vi "Basic_pn_SH.vi"(7 "BitFile Path":string="C:\\Users\\kalyan\\Desktop\\5775_digitizer\\Host\\PXIe_5775_KU035.lvbitx", 9 "AI num samples":u64=320 step=16, 10 "AI channels":string="AI0,AI1", 11 "Device Id":string="PXI1Slot5") -> (0 "error out":errorcluster, 1 "dt":dbl, 2 "SecondChannel":dbl[](array[numeric]), 3 "FirstChannel":dbl[](array[numeric]))   [LabVIEW 2019, in "GettingStarted_5775_Host.lvlib"]
uses:
  GettingStarted_5775_Host.lvlib
  <instrlib>/FlexRIO/API/Host/v1/NI FlexRIO/API/Reference Clock Source.ctl
  <instrlib>/FlexRIO/API/Host/v1/NI FlexRIO/API/Configure Reference Clock.vi
  <instrlib>/FlexRIO/API/Host/v1/NI FlexRIO/API/Get Property Reference - Fpga Small.vi
  <instrlib>/FlexRIO/API/Host/v1/NI FlexRIO/API/Configure Analog Start Trigger.vi
  <instrlib>/FlexRIO/API/Host/v1/NI FlexRIO/API/Configure Digital Edge Start Trigger.vi
  <instrlib>/FlexRIO/API/Host/v1/NI FlexRIO/API/Configure Immediate Start Trigger.vi
  <instrlib>/FlexRIO/API/Host/v1/NI FlexRIO/API/Read Stream 2D F64.vi
  <vilib>/FPGAPlugInAG/Dynamic/niLvFpga_Close_Dynamic.vi
  <vilib>/rvi/interface/nirviCloseFPGA/nirviCloseFPGA.xnode
  <instrlib>/FlexRIO/API/Host/v1/NI FlexRIO API v1.lvlib
  <resource>/objmgr/niflexrioapiStream.rc
panel:
  out "numSamples":i32
  in  "reference clock source":T1 items=["Default", "Onboard", "PXI_Clk10", "External", "None", "Baseboard Reference"]
  out "Acquisition time":dbl=3200000000.0 format="%#_6p"
  in  "ADC Interleaving Factor":i32=1 min=0 max=2 step=1
  out "Device Power":dbl(slide) scale=-1.0..38.0 scale format="%#_3p"
  out "FPGA Temperature":dbl(slide) scale=0.0..100.0 scale format="%#_3p"
  in  "Trigger Type":enum32{"Immediate", "Analog", "Digital"}(tab)
  in  "trigger channel":string="AI0"
  in  "rising edge?":bool=TRUE
  in  "level (V)":dbl format="%#_3p"
  in  "hysteresis (V)":dbl format="%#_3p"
  in  "digital trigger source":string(combo)
  in  "Waveform Tab Control":enum32{"AI Time Domain", "AI Frequency Domain"}(tab)
  out "Waveform Graph":dbl[][](graph)
  out "Limit (W)":dbl
  out "Power (W)":dbl
  out "Limit (C)":dbl
  out "Temp (C)":dbl format="%#_4p"
  # "Overview: Configure an acquisition for a FlexRIO target and transfer the data to the host using the FlexRIO Host API.  Loop an output waveform\nRequirements: FlexRIO\nInstructions: \n 1. Select the RIO Device that corresponds to the FlexRIO target. \n 2. Select the bitfile path that corresponds to your device\n 3. Optionally configure the clocking, stream, and trigger. \n 4. Run the VI"
  # "Resource Configuration"
  # "Clocking configuration"
  # "Input Waveform Configuration"
  # "Device Monitoring"
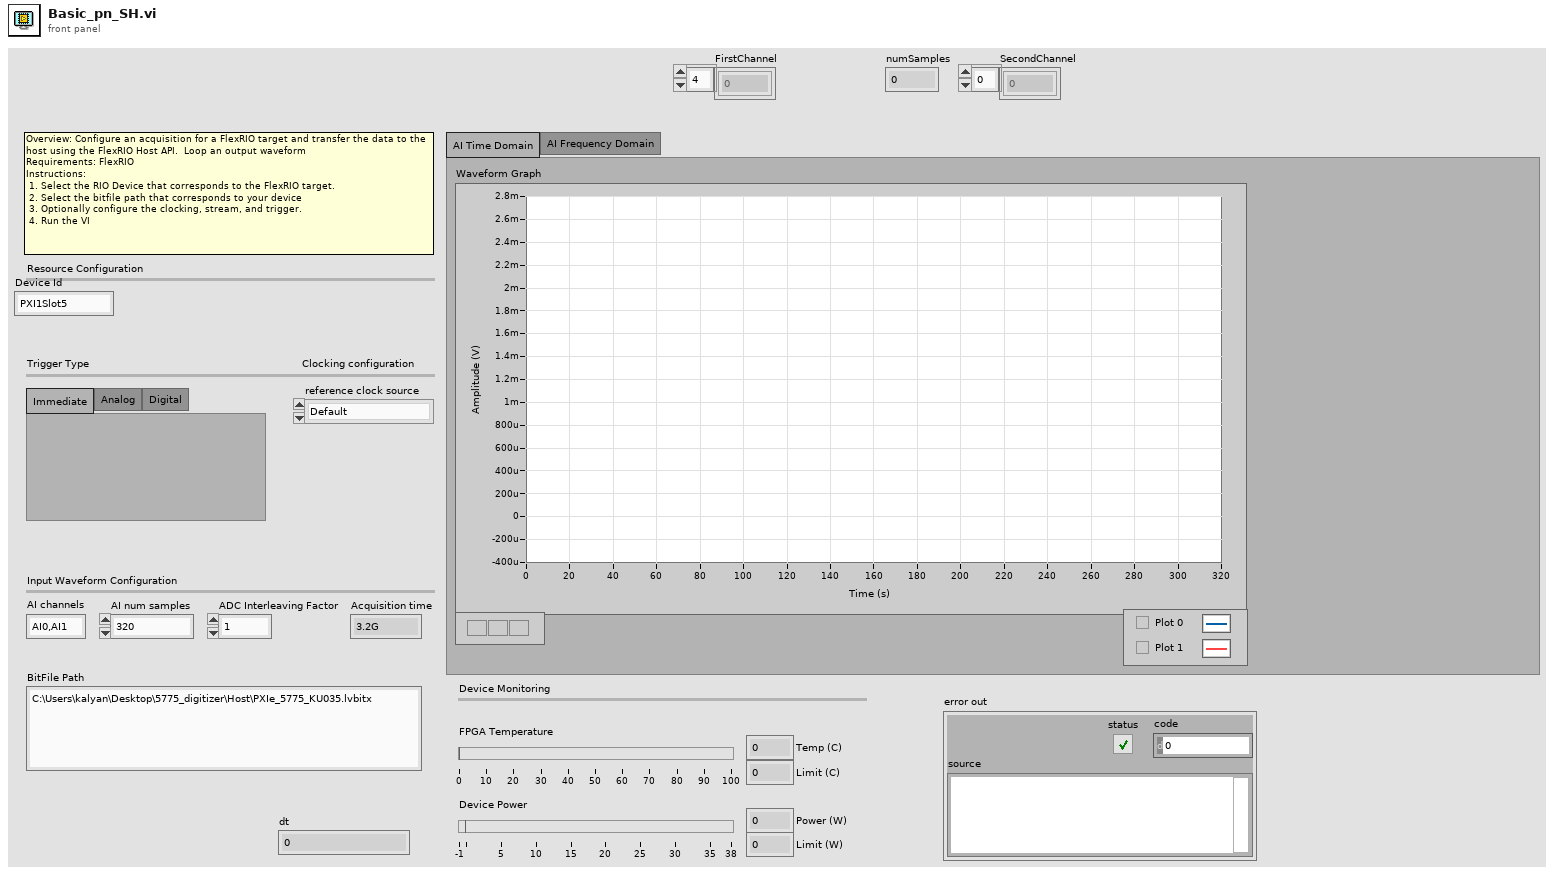
[diagram p1: front panel]
types:
  T1 = typedef "NI FlexRIO API v1.lvlib/Reference Clock Source.ctl" = i32
  T2 = typedef "NI FlexRIO API v1.lvlib/Waveform Info.ctl" = cluster{"absoluteInitialXUpper":dbl, "absoluteInitialXLower":dbl, "relativeInitialX":dbl, "dt":dbl, "gain":dbl, "offset":dbl, "reserved 1":dbl, "reserved 2":dbl, "# of elements":u64, "reserved 3":u64}
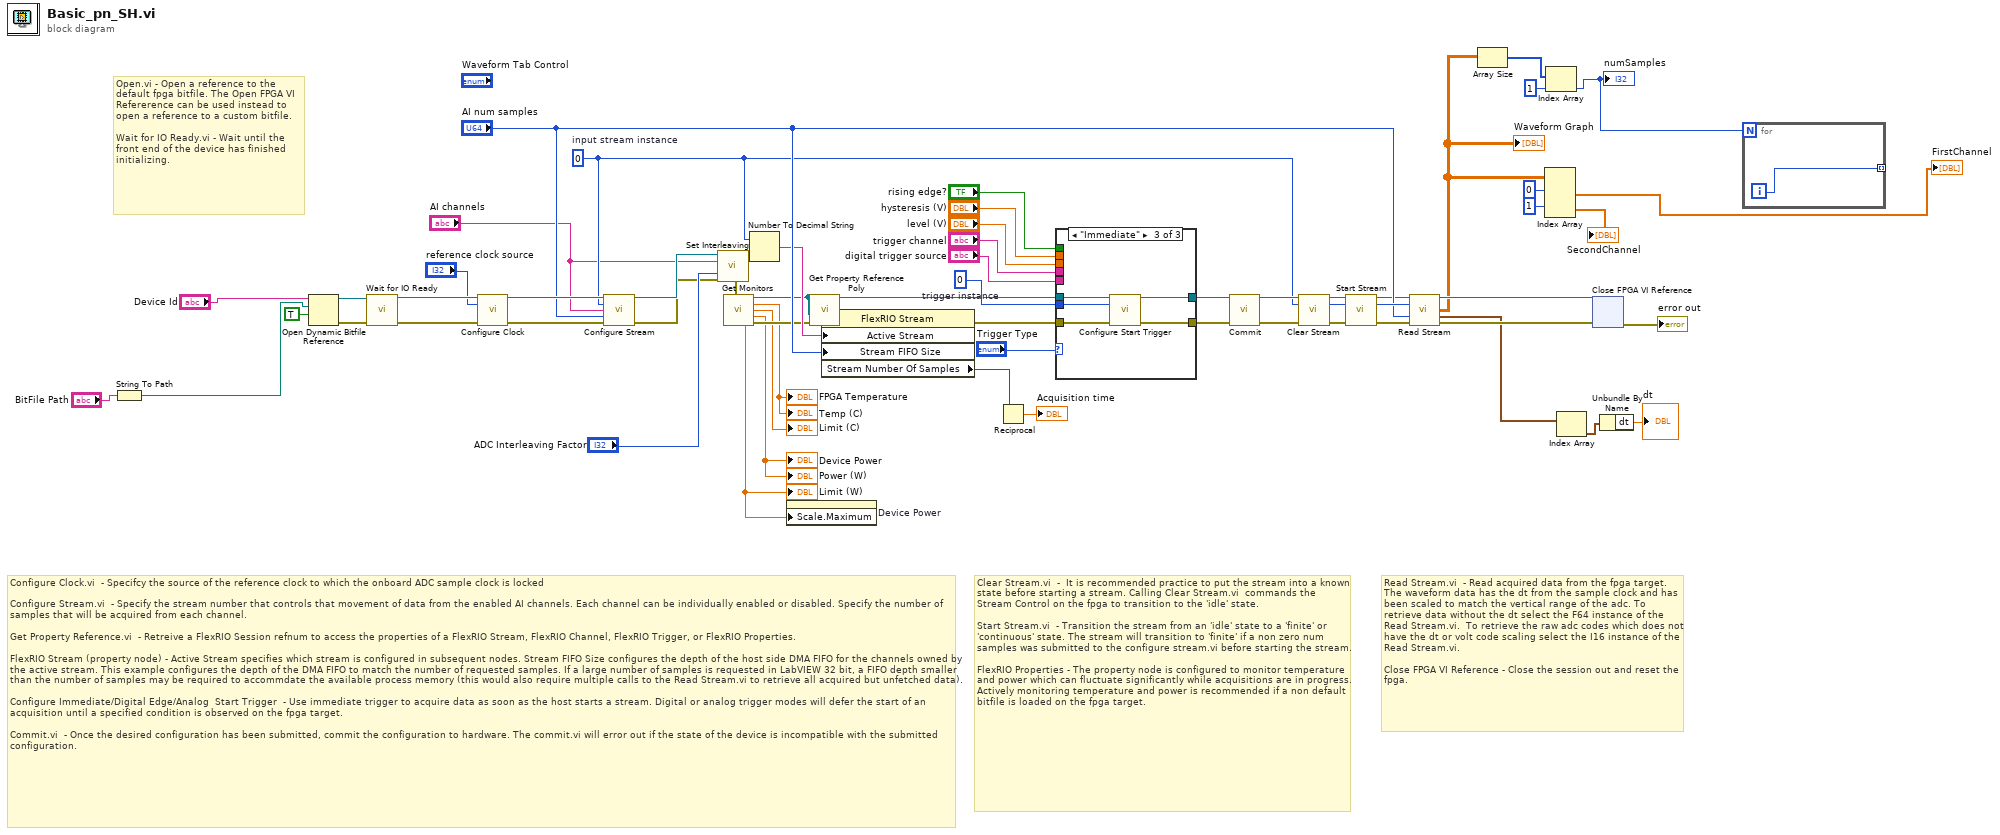
[diagram p0: block diagram]
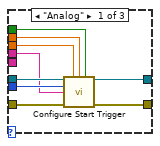
[diagram p2: hidden frame]
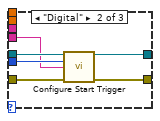
[diagram p3: hidden frame]
diagram:
  w42 = u32 0  # trigger instance
  w33 = u32 0  # input stream instance
  # "Read Stream.vi  - Read acquired data from the fpga target. The waveform data has the dt from the sample clock and has been scaled to match the vertical range of the adc. To retrieve data without the dt select the F64 instance of the Read Stream.vi.  To retrieve the raw adc codes which does not have the dt or volt code scaling select the I16 instance of the Read Stream.vi.  \n\nClose FPGA VI Reference - Close the session out and reset the fpga."
  # "Clear Stream.vi  -  It is recommended practice to put the stream into a known state before starting a stream. Calling Clear Stream.vi  commands the Stream Control on the fpga to transition to the 'idle' state.\n\nStart Stream.vi  - Transition the stream from an 'idle' state to a 'finite' or 'continuous' state. The stream will transition to 'finite' if a non zero num samples was submitted to the configure stream.vi before starting the stream.  \n\nFlexRIO Properties - The property node is configured to monitor temperature and power which can fluctuate significantly while acquisitions are in progress. Actively monitoring temperature and power is recommended if a non default bitfile is loaded on the fpga target."
  # "Configure Clock.vi  - Specifcy the source of the reference clock to which the onboard ADC sample clock is locked\n\nConfigure Stream.vi  - Specify the stream number that controls that movement of data from the enabled AI channels. Each channel can be individually enabled or disabled. Specify the number of samples that will be acquired from each channel. \n\nGet Property Reference.vi  - Retreive a FlexRIO Session refnum to access the properties of a FlexRIO Stream, FlexRIO Channel, FlexRIO Trigger, or FlexRIO Properties.\n\nFlexRIO Stream (property node) - Active Stream specifies which stream is configured in subsequent nodes. Stream FIFO Size configures the depth of the host side DMA FIFO for the channels owned by the active stream. This example configures the depth of the DMA FIFO to match the number of requested samples. If a large number of samples is requested in LabVIEW 32 bit, a FIFO depth smaller than the number of samples may be required to accommdate the available process memory (this would also require multiple calls to the Read Stream.vi to retrieve all acquired but unfetched data). \n\nConfigure Immediate/Digital Edge/Analog  Start Trigger  - Use immediate trigger to acquire data as soon as the host starts a stream. Digital or analog trigger modes will defer the start of an acquisition until a specified condition is observed on the fpga target. \n\nCommit.vi  - Once the desired configuration has been submitted, commit the configuration to hardware. The commit.vi will error out if the state of the device is incompatible with the submitted configuration."
  # "Open.vi - Open a reference to the default fpga bitfile. The Open FPGA VI Refererence can be used instead to open a reference to a custom bitfile.\n\nWait for IO Ready.vi - Wait until the front end of the device has finished initializing."
  n1 = String To Path(string="BitFile Path") -> (path=w2:path)
  n2 = Open Dynamic Bitfile Reference(0:"Device Id", 1:w2, 2:TRUE ("Run When Loaded")) -> (5:w58:refnum<k20>, 8:w59:errorcluster)  [unwired: 2 in]
  n3 = call <instrlib>:"Wait for IO Ready.vi"("fpga interface in"=w58, "error in"=w59) -> ("fpga interface out"=w60:refnum<k20>, "error out"=w61:errorcluster)  [unwired: 10 in, 2 out]
  n4 = call-poly <instrlib>:"Configure Clock.vi"("fpga interface in"=w60, "reference clock source"="reference clock source", "error in"=w61) -> ("fpga interface out"=w48:refnum<k20>, "error out"=w47:errorcluster)  [unwired: 11 in]
  n5 = call <instrlib>:"Configure Stream.vi"("fpga interface in"=w48, "stream instance"=w33, "channels enabled"="AI channels", "num samples"="AI num samples", "error in"=w47) -> ("fpga interface out"=w28:refnum<k20>, "error out"=w26:errorcluster)  [unwired: 7 in, 2 out]
  n6 = call "Set Interleaving.vi"("fpga interface in"=w28, "AI channels enabled"="AI channels", "ADC Interleaving Factor"="ADC Interleaving Factor", "error in (no error)"=w26) -> ("fpga interface out"=w29:refnum<k20>, "error out"=w30:errorcluster)  [unwired: 10 in]
  n7 = call "Get Monitors.vi"("fpga interface in"=w29, "error in (no error)"=w30) -> ("fpga interface out"=w22:refnum<k20>, "FPGA Temperature (C)"=→"Temp (C)" →"FPGA Temperature":dbl, "Temperature Limit (C)"=→"Limit (C)":dbl, "Total Power (W)"=→"Power (W)" →"Device Power":dbl, "Power Limit (W)"=w18:dbl, "error out"=w25:errorcluster)  [unwired: 8 in]
  "Limit (W)" <- w18
  n8 = Number To Decimal String(number=w33) -> (decimal integer string=w44:string)  [unwired: 1 in]
  n9 = property on="Device Power" class="Slide (strict)"("Scale.Maximum"=w18) -> ()  [unwired: 2 in, 2 out]
  n10 = call-poly <instrlib>:"Get Property Reference Poly.vi"("error in (no error)"=w25, "fpga interface in"=w22) -> ("error out"=w24:errorcluster, "property reference"=w23:refnum<k20>)  [unwired: 4 in, 1 out]
  n11 = property class="FlexRIO Stream"(reference=w23, error in=w24, "Active Stream"=w44, "Stream FIFO Size"="AI num samples") -> (error out=w39:errorcluster, "Stream Number Of Samples"=w32:u64)  [unwired: 1 out]
  n12 = Reciprocal(x=w32) -> (1/x=→"Acquisition time":dbl)
  n13 = case shown="\"Immediate\"" "Trigger Type" {
    tunnel: w22 -> [w71 w77 w82]
    tunnel: w39 -> [w70 w76 w81]
    tunnel: [w69 w75 w80] -> w38
    tunnel: [w68 w74 w79] -> w37
    tunnel: w42 -> [w67 w73 w78]
    tunnel: "trigger channel" -> [w66 _ _]
    tunnel: "level (V)" -> [w65 _ _]
    tunnel: "hysteresis (V)" -> [w64 _ _]
    tunnel: "rising edge?" -> [w63 _ _]
    tunnel: "digital trigger source" -> [_ w72 _]
    frame "Analog" {
      n14 = call-poly <instrlib>:"Configure Start Trigger.vi"("fpga interface in"=w71, "level"=w65, "hysteresis"=w64, "rising edge?"=w63, "trigger instance"=w67, "channel"=w66, "error in"=w70) -> ("fpga interface out"=w69:refnum<k20>, "error out"=w68:errorcluster)  [unwired: 6 in, 1 out]
    }
    frame "Digital" {
      n15 = call-poly <instrlib>:"Configure Start Trigger.vi"("fpga interface in"=w77, "trigger instance"=w73, "trigger source"=w72, "error in"=w76) -> ("fpga interface out"=w75:refnum<k20>, "error out"=w74:errorcluster)  [unwired: 9 in, 1 out]
    }
    frame "Immediate" {
      n16 = call-poly <instrlib>:"Configure Start Trigger.vi"("fpga interface in"=w82, "trigger instance"=w78, "error in"=w81) -> ("fpga interface out"=w80:refnum<k20>, "error out"=w79:errorcluster)  [unwired: 10 in, 1 out]
    }
  }
  n17 = call <instrlib>:"Commit.vi"("fpga interface in"=w38, "error in"=w37) -> ("fpga interface out"=w41:refnum<k20>, "error out"=w34:errorcluster)  [unwired: 12 in]
  n18 = call <instrlib>:"Clear Stream.vi"("fpga interface in"=w41, "stream instance"=w33, "error in"=w34) -> ("fpga interface out"=w51:refnum<k20>, "stream instance out"=w50:u32, "error out"=w49:errorcluster)  [unwired: 10 in]
  n19 = call <instrlib>:"Start Stream.vi"("fpga interface in"=w51, "stream instance"=w50, "error in"=w49) -> ("fpga interface out"=w36:refnum<k20>, "stream instance out"=w46:u32, "error out"=w35:errorcluster)  [unwired: 10 in]
  n20 = call-poly <instrlib>:"Read Stream.vi"("fpga interface in"=w36, "stream instance"=w46, "samples"="AI num samples", "error in"=w35) -> ("fpga interface out"=w56:refnum<k20>, "read data"=w9:dbl[][], "wfm info"=w13:T2[], "error out"=w15:errorcluster)  [unwired: 7 in, 1 out]
  "Waveform Graph" <- w9
  n21 = Array Size(array=w9) -> (size(s)=w11:i32[])
  n22 = Index Array(array=w9, index (row) #1=0 ("index (row)"), index (row) #2=1 ("index (row)")) -> (element #1=→"FirstChannel":dbl[], element #2=→"SecondChannel":dbl[])  [unwired: 2 in]
  n23 = Index Array(array=w11, index=1) -> (element=w4:i32)
  "numSamples" <- w4
  n24 = Index Array(array=w13) -> (element=w12:T2)  [unwired: 1 in]
  n25 = xnode "Close FPGA VI Reference"("FPGA VI Reference In"=w56, "error in"=w15) -> ("error out"=→"error out":errorcluster)
  n26 = Unbundle By Name(w12) -> ("dt"=→"dt":dbl)
  n27 = for {
    N: w4 -> [_]
    tunnel: [w83] -> _ mode=indexing
    i -> [w83]
  }
